vi "GEOM_VAR_FPA2.vi"(9 "Action":T9, 10 "GEOM_FPA":T8 {"Sorted Detectors"."ReadModes"."amplifiers"."fliped" items=["none", "horizontal", "vertical"]; "Sorted Detectors"."ReadModes"."amplifiers"."type" items=["LL", "LR", "UL", "UR"]}) -> (2 "GEOM_FPA out":T8 {"Sorted Detectors"."ReadModes"."amplifiers"."fliped" items=["none", "horizontal", "vertical"]; "Sorted Detectors"."ReadModes"."amplifiers"."type" items=["LL", "LR", "UL", "UR"]})   [LabVIEW 2016]
uses:
  GEOM_VAR_action.ctl
  GEOM_FPADetectors.ctl
  GEOM_DetStruct.ctl
  GEOM_ReadMode.ctl
  GEOM_Amplifier.ctl
  GEOM_AmpType.ctl
  GEOM_ROI.ctl
  GEOM_Coords.ctl
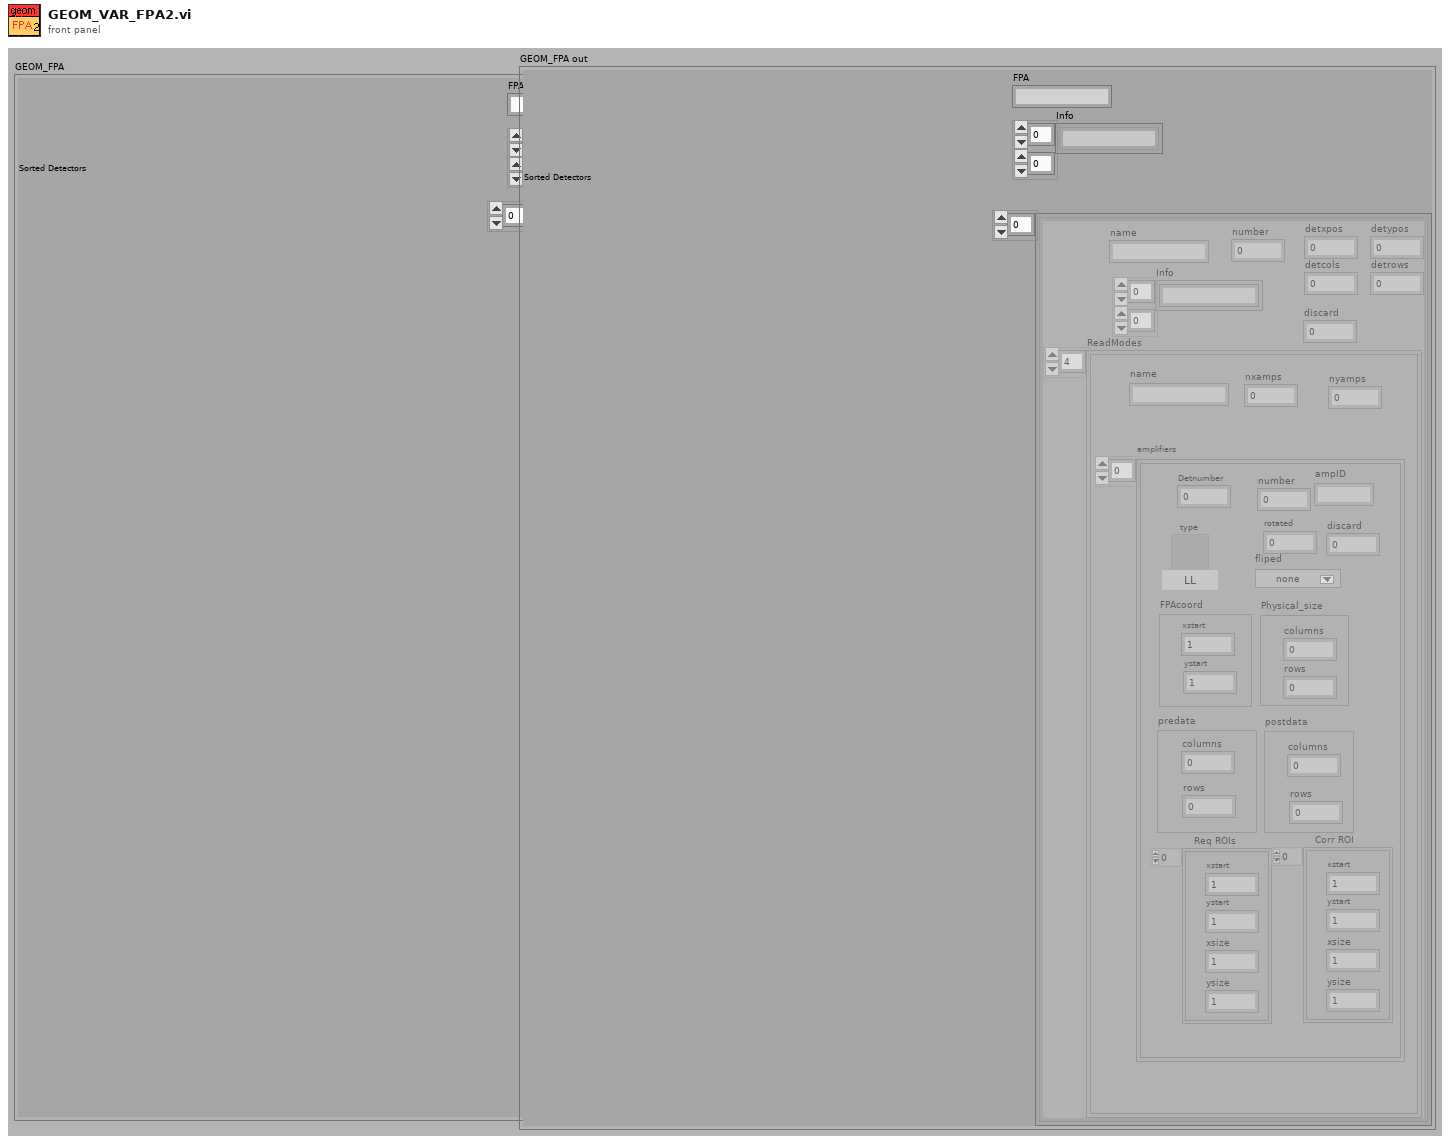
[diagram p1: front panel]
types:
  T1 = typedef "GEOM_FPADetectors.ctl" = T2[]
  T2 = typedef "GEOM_DetStruct.ctl" = cluster{"name":string, "number":i32, "Info":string[][], "ReadModes":T3[], "detxpos":i32, "detypos":i32, "detcols":i32, "detrows":i32, "discard":i32}
  T3 = typedef "GEOM_ReadMode.ctl" = cluster{"name":string, "amplifiers":T4[], "nxamps":i32, "nyamps":i32}
  T4 = typedef "GEOM_Amplifier.ctl" = cluster{"number":i32, "type":T5, "rotated":i16, "fliped":u16, "FPAcoord":cluster{"xstart":i32, "ystart":i32}, "Physical_size":cluster{"columns":i32, "rows":i32}, "predata":cluster{"columns":i32, "rows":i32}, "postdata":cluster{"columns":i32, "rows":i32}, "Req ROIs":T6, "Corr ROI":T6, "Detnumber":i32, "ampID":string, "discard":i32}
  T5 = typedef "GEOM_AmpType.ctl" = u16
  T6 = typedef "GEOM_ROI.ctl" = T7[]
  T7 = typedef "GEOM_Coords.ctl" = cluster{"xstart":u32, "ystart":u32, "xsize":u32, "ysize":u32}
  T8 = cluster{"FPA":string, "Info":string[][], "Sorted Detectors":T1}
  T9 = typedef "GEOM_VAR_action.ctl" = enum16{"read", "write"}
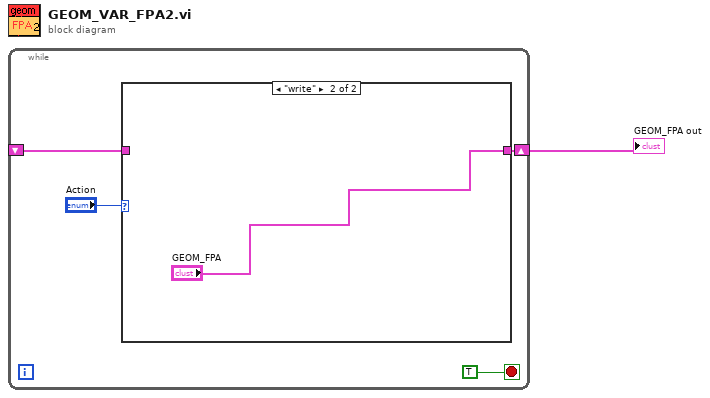
[diagram p0: block diagram]
diagram:
  n1 = while {
    shift-right: [w4] -> w1
    shift-left: _ -> [w3]
    stop <- TRUE stop-if-true
    n2 = case shown="\"write\"" "Action" {
      tunnel: [w6 "GEOM_FPA"] -> w4
      tunnel: w3 -> [w6 _]
      frame "read", Default {
      }
      frame "write" {
      }
    }
  }
  "GEOM_FPA out" <- w1
